vi "LIN_Demo_Template.vi"() -> ()   [LabVIEW 2014]
uses:
  TSMaster_API/All_Control/Typedef/Hardware Type.ctl
  Utilities/Typedef/Hardware_Subtype.ctl
  TSMaster_API/LIN_Function/Typedef/TSLIN_SetData.ctl
  TSMaster_API/LIN_Function/Typedef/TSLIN_Transmit.ctl
  TSMaster_API/LIN_Function/Typedef/TLibLIN.ctl
panel:
  out "ALINBuffer":T1[](array[typedef]) {"ID" format="%x"}
  # "使用方法：\n1.创建TSMaster 工程，映射通道2，并开启接收Trace\n2.此demo 映射通道1\n3.通道1与通道2进行短接\n4.运行此demo 发送Fdata ,并接收Fdata"
  # "usage method:\n1. Create TSMaster project, map channel\n2, and enable receiving Trace. 2. This demo maps channel 1. \n3. Short circuit channel 1 to channel 2\n4. Run this demo sends and receives Fdata"
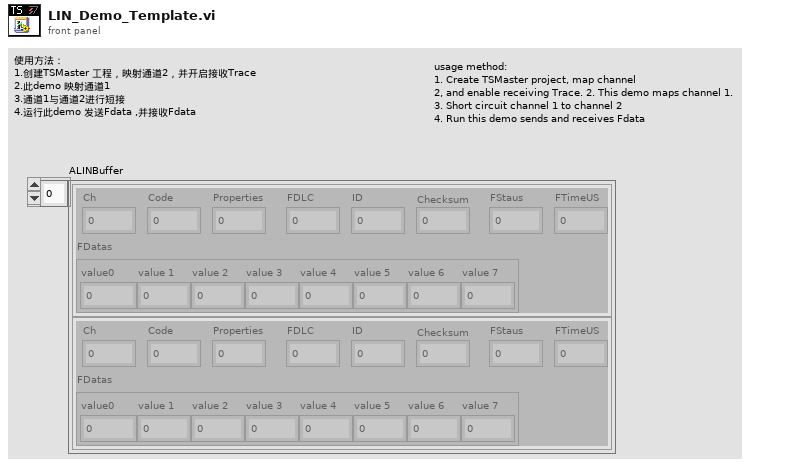
[diagram p1: front panel]
types:
  T1 = typedef "TLibLIN.ctl" = cluster{"Ch":u8, "Code":u8, "Properties":u8, "FDLC":u8, "ID":u8, "Checksum":u8, "FStaus":u8, "FTimeUS":u64, "FDatas":cluster{"value0":u8, "value 1":u8, "value 2":u8, "value 3":u8, "value 4":u8, "value 5":u8, "value 6":u8, "value 7":u8}}
  T2 = enum16{"Only read received messages", "Receive&send messages"}
  T3 = typedef "TSLIN_SetData.ctl" = cluster{"Hardware Type":T4, "Hardware Subtype":T5, "AHwChannel":i32, "AAppChannel":i32, "ABaudrateKbps":sgl, "AProtocol":i32, "AldHW":i32}
  T4 = typedef "Hardware Type.ctl" = i32
  T5 = typedef "Hardware_Subtype.ctl" = enum16{"TS_UNKNOWN_DEVICE", "TSCAN_PRO", "TSCAN_Lite1", "TC1001", "TL1001", "TC1011", "TM5011", "TC1002", "TC1014", "TSCANFD2517", "TC1026", "TC1016", "TC1012", "TC1013", "TLog1002", "TC1034", "TC1018", "GW2116", "TC2115", "MP1013", "TC1113", "TC1114", "TP1013", "TC1017", "TP1018", "TF10XX", "TL1004_FD_4_LIN_2", "TE1051", "TP1051", "TP1034", "TTS9015", "TP1026", "TTS1026", "TTS1034", "TTS1018", "TL1011", "TTS1015_LiAuto", "TTS1013_LiAuto", "TTS1016Pro", "TC1054Pro", "TC1054", "TLog1038", "TO1013", "TC1034Pro", "TC1018Pro", "TC1038Pro", "TS_DEV_END"}
  T6 = typedef "TSLIN_Transmit.ctl" = cluster{"Channel":i32, "Rx/TX":enum16{"Rx", "Tx"}, "Set_node_funtiontype":i32, "DLC":u32, "ID":u32, "FDatas":cluster{"value0":u8, "value 1":u8, "value 2":u8, "value 3":u8, "value 4":u8, "value 5":u8, "value 6":u8, "value 7":u8}}
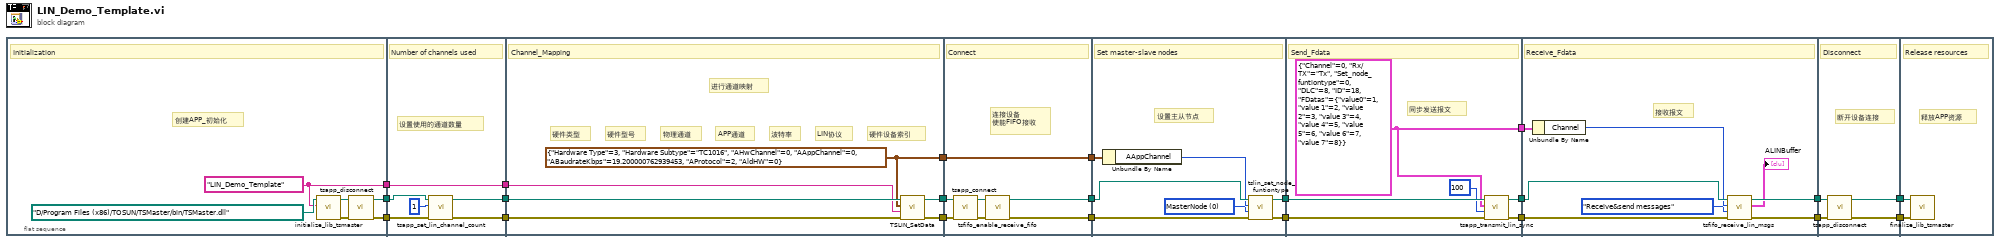
[diagram p0: block diagram]
diagram:
  n1 = flat-sequence {
    tunnel: [w24] -> w21
    tunnel: [w23] -> w20
    tunnel: [w22] -> w16
    tunnel: w21 -> [w33]
    tunnel: w20 -> [w32]
    tunnel: [w30] -> w19
    tunnel: [w29] -> w18
    tunnel: [w28] -> w17
    tunnel: w16 -> [w28]
    tunnel: w19 -> [w39]
    tunnel: w18 -> [w38]
    tunnel: w17 -> [w37]
    tunnel: [w36] -> w15
    tunnel: [w35] -> w14
    tunnel: [w34] -> w11
    tunnel: w15 -> [w45]
    tunnel: w14 -> [w43]
    tunnel: [w42] -> w13
    tunnel: [w41] -> w12
    tunnel: w11 -> [w40]
    tunnel: [w40] -> w10
    tunnel: w13 -> [w53]
    tunnel: w12 -> [w52]
    tunnel: w10 -> [w51]
    tunnel: [w48] -> w9
    tunnel: [w47] -> w8
    tunnel: w9 -> [w59]
    tunnel: w8 -> [w58]
    tunnel: [w56] -> w7
    tunnel: [w55] -> w6
    tunnel: [w54] -> w5
    tunnel: w7 -> [w67]
    tunnel: w6 -> [w66]
    tunnel: w5 -> [w65]
    tunnel: [w62] -> w4
    tunnel: [w61] -> w3
    tunnel: w4 -> [w71]
    tunnel: w3 -> [w70]
    tunnel: [w69] -> w2
    tunnel: [w68] -> w1
    tunnel: w2 -> [w73]
    tunnel: w1 -> [w72]
    frame #0 {
      w22 = "LIN_Demo_Template" ("AppName")
      # "创建APP_初始化"
      # "Initialization"
      n2 = call "initialize_lib_tsmaster.vi"("AppName"=w22, "Path input"=path "D:/Program Files (x86)/TOSUN/TSMaster/bin/TSMaster.dll") -> ("error output"=w27:errorcluster, "Path output"=w26:path)  [unwired: 8 in]
      n3 = call "tsapp_disconnect.vi"("error in (no error)"=w27, "Path"=w26) -> ("error output"=w23:errorcluster, "Path output"=w24:path)  [unwired: 7 in, 1 out]
    }
    frame #1 {
      # "设置使用的通道数量"
      # "Number of channels used"
      n4 = call "tsapp_set_lin_channel_count.vi"("error in (no error)"=w32, "Aount"=1, "Path"=w33) -> ("error out"=w29:errorcluster, "Path output"=w30:path)  [unwired: 6 in, 1 out]
    }
    frame #2 {
      w34 = T3 {"Hardware Type"=3, "Hardware Subtype"=enum."TC1016", "AHwChannel"=0, "AAppChannel"=0, "ABaudrateKbps"=19.2, "AProtocol"=2, "AldHW"=0} ("Set")
      # "硬件设备索引"
      # "LIN协议"
      # "波特率"
      # "APP通道"
      # "物理通道"
      # "硬件型号"
      # "硬件类型"
      # "进行通道映射"
      # "Channel_Mapping"
      n5 = call "TSLIN_SetData.vi"("Error in"=w38, "AppName"=w37, "Set"=w34, "Path"=w39) -> ("Error out"=w35:errorcluster, "Path output"=w36:path)  [unwired: 4 in, 2 out]
    }
    frame #3 {
      # "连接设备\n使能FIFO接收"
      # "Connect"
      n6 = call "tsapp_connect.vi"("error in (no error)"=w43, "Path"=w45) -> ("error out"=w46:errorcluster, "Path output"=w44:path)  [unwired: 7 in, 1 out]
      n7 = call "tsfifo_enable_receive_fifo.vi"("error in (no error)"=w46, "Path"=w44) -> ("error out"=w41:errorcluster, "Path output"=w42:path)  [unwired: 8 in]
    }
    frame #4 {
      w49 = 0 items=["MasterNode", "SlaveNode", "MonitorNote"] ("set_node_funtiontype")
      # "设置主从节点"
      # "Set master-slave nodes"
      n8 = Unbundle By Name(w51) -> ("AAppChannel"=w50:i32)
      n9 = call "tslin_set_node_funtiontype.vi"("错误输入（无错误）"=w52, "set_node_funtiontype"=w49, "AAppChannel"=w50, "path"=w53) -> ("错误输出"=w47:errorcluster, "path out"=w48:path)  [unwired: 5 in, 1 out]
    }
    frame #5 {
      w54 = T6 {"Channel"=0, "Rx/TX"=enum."Tx", "Set_node_funtiontype"=0, "DLC"=8, "ID"=18, "FDatas"={"value0"=1, "value 1"=2, "value 2"=3, "value 3"=4, "value 4"=5, "value 5"=6, "value 6"=7, "value 7"=8}} ("LIN_Transmit")
      # "同步发送报文"
      # "Send_Fdata"
      n10 = call "tsapp_transmit_lin_sync.vi"("错误输入（无错误）"=w58, "ATimeoutMS"=100, "LIN_Transmit"=w54, "路径输入"=w59) -> ("错误输出"=w55:errorcluster, "路径输出"=w56:path)  [unwired: 5 in, 1 out]
    }
    frame #6 {
      # "接收报文"
      # "Receive_Fdata"
      n11 = Unbundle By Name(w65) -> ("Channel"=w64:i32)
      n12 = call "tsfifo_receive_lin_msgs.vi"("错误输入（无错误）"=w66, "Read message type"=T2."Receive&send messages", "AIdxChn"=w64, "路径输入"=w67) -> ("错误输出"=w61:errorcluster, "ALINBuffer"=→"ALINBuffer":T1[], "路径输出"=w62:path)  [unwired: 4 in, 1 out]
    }
    frame #7 {
      # "断开设备连接"
      # "Disconnect"
      n13 = call "tsapp_disconnect.vi"("error in (no error)"=w70, "Path"=w71) -> ("error output"=w69:errorcluster, "Path output"=w68:path)  [unwired: 7 in, 1 out]
    }
    frame #8 {
      # "释放APP资源"
      # "Release resources"
      n14 = call "finalize_lib_tsmaster.vi"("error in (no error)"=w73, "Path"=w72) -> ()  [unwired: 8 in, 2 out]
    }
  }
